vi "input_vel.vi"(3 "error in (no error)":errorcluster, 4 "input":dbl, 5 "odrive":refnum<visa-resource-name>) -> (0 "error out":errorcluster, 1 "String":string, 2 "VISA resource name out":refnum<visa-resource-name>)   [LabVIEW 2019]
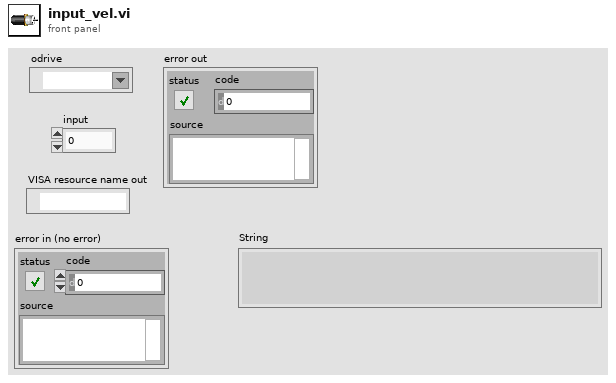
[diagram p1: front panel]
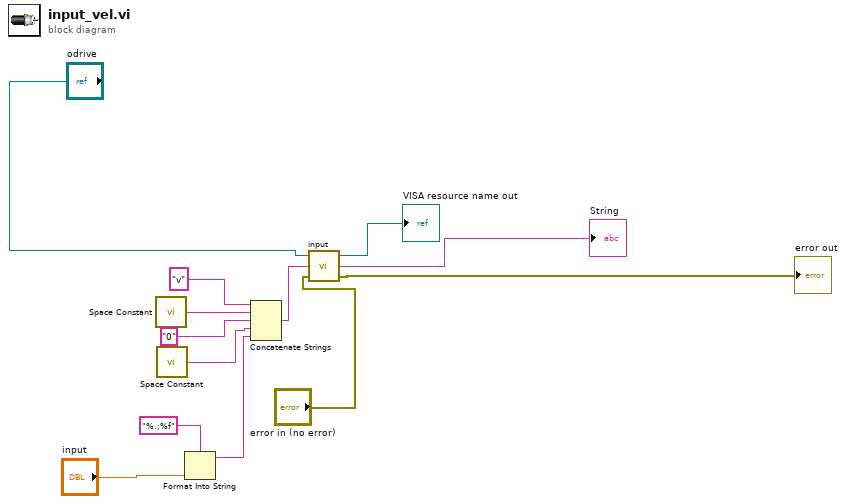
[diagram p0: block diagram]
diagram:
  n1 = call <vilib>:"Space Constant.vi"() -> ("String"=w11:string)
  n2 = call <vilib>:"Space Constant.vi"() -> ("String"=w13:string)
  n3 = Format Into String(format string="%.;%f", "input") -> (resulting string=w7:string)  [unwired: 2 in, 1 out]
  n4 = Concatenate Strings("v" ("write buffer"), w11, "0", w13, w7) -> (w2:string)
  n5 = call "input.vi"("error in (no error)"="error in (no error)", "commando"=w2, "VISA in"="odrive") -> ("error out"=→"error out":errorcluster, "DEBUG"=→"String":string, "VISA out"=→"VISA resource name out":refnum<visa-resource-name>)
